vi "getLVProjBuildItems(From XML).vi"(8 "error in (no error)":errorcluster, 11 "Path":path=path "Y:/Dossiers Personnels/BRO/DevTools_BR/BuildAutomation/Builder/Builder.lvproj") -> (0 "error out":errorcluster, 1 "BuildSpec Names":string[][](array[string]), 2 "Target Names":string[](array[string]), 3 "Project Name":string, 4 "BuildSpec Types":string[][](array[string]), 5 "Project Path":path=path "Y:/Dossiers Personnels/BRO/DevTools_BR/BuildAutomation/Builder/Builder.lvproj")   [LabVIEW 2017, in "BuildServer.lvlib" / "BuildServer.lvclass"]
uses:
  BuildServer.lvclass
  <vilib>/xml/Load XML File.vi
  <vilib>/xml/Close Reference(Node).vi
  <vilib>/xml/Close Reference(NNMap).vi
  <vilib>/xml/NI_XML.lvlib
  <resource>/objmgr/DOMUserDefRef.rc
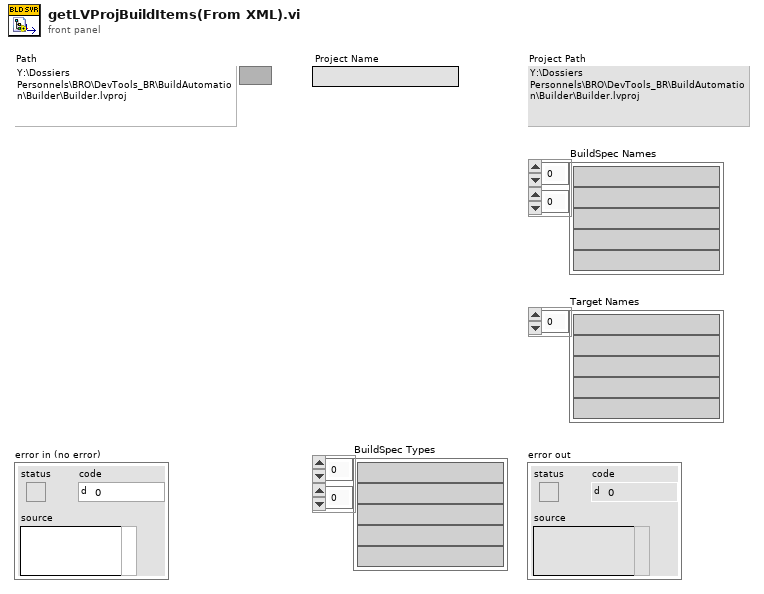
[diagram p1: front panel]
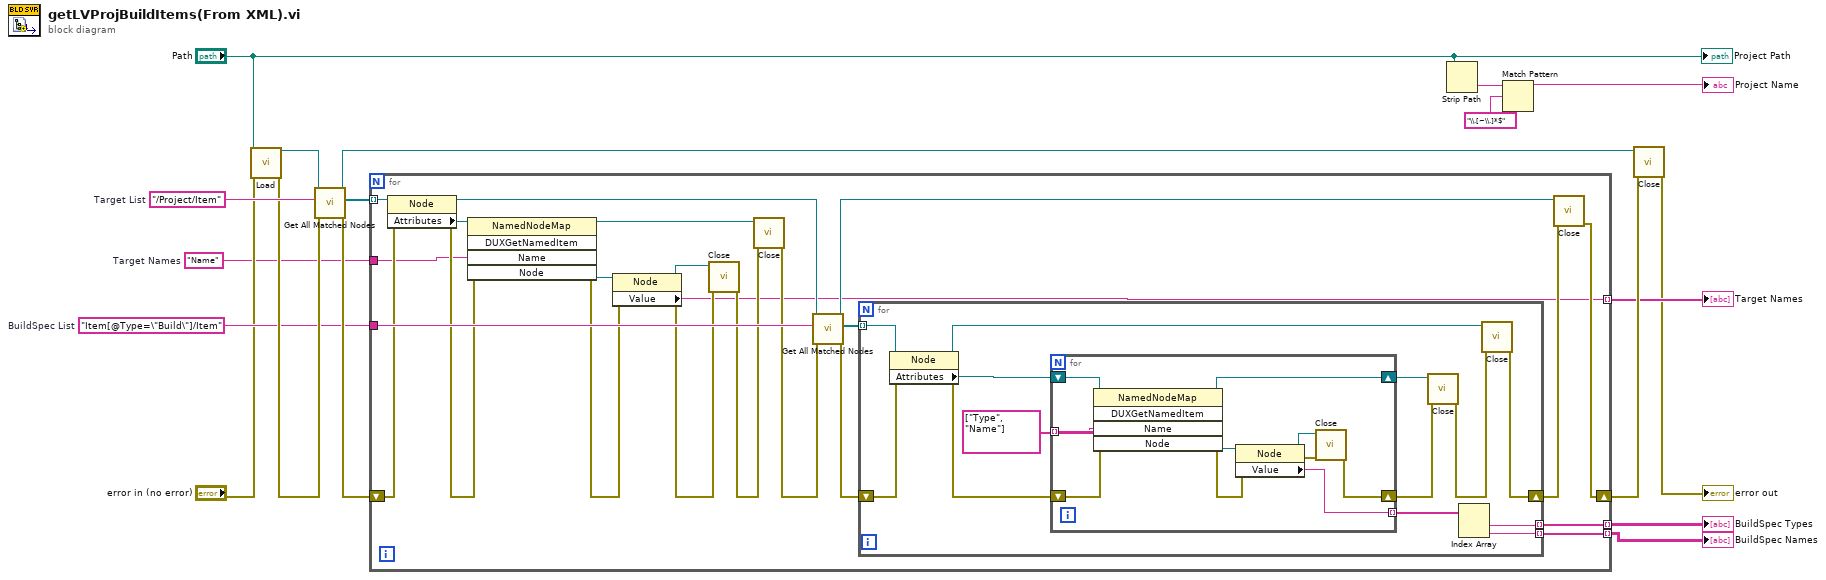
[diagram p0: block diagram]
diagram:
  w7 = "Name"  # Target Names
  w13 = "Item[@Type=\"Build\"]/Item"  # BuildSpec List
  w17 = "/Project/Item"  # Target List
  n1 = call-poly <vilib>:"Load.vi"("path to XML document"="Path", "error in (no error)"="error in (no error)") -> ("DOM document out"=w18:refnum<k20>, "error out"=w16:errorcluster)  [unwired: 11 in, 1 out]
  n2 = call <vilib>:"Get All Matched Nodes.vi"("error in (no error)"=w16, "XPath expression"=w17, "node in"=w18) -> ("error out"=w14:errorcluster, "node result array"=w15:refnum<k20>[], "node out"=w12:refnum<k20>)  [unwired: 6 in]
  n3 = for {
    tunnel: w15 -> [w34] mode=indexing
    shift-right: [w35] -> w11
    shift-left: w14 -> [w26]
    tunnel: w13 -> [w36]
    tunnel: [w22] -> w10 mode=indexing
    tunnel: w7 -> [w21]
    tunnel: [w20] -> w5 mode=indexing
    tunnel: [w19] -> w4 mode=indexing
    n4 = property class="Node"(reference=w34, error in=w26) -> (reference out=w33:refnum<k20>, error out=w27:errorcluster, "Attributes"=w32:refnum<k20>)
    n5 = invoke class="NamedNodeMap" method="DUXGetNamedItem"(reference=w32, error in=w27, "Name"=w21) -> (reference out=w25:refnum<k20>, error out=w28:errorcluster, "Node"=w31:refnum<k20>)  [unwired: 2 in, 2 out]
    n6 = property class="Node"(reference=w31, error in=w28) -> (reference out=w30:refnum<k20>, error out=w29:errorcluster, "Value"=w22:string)
    n7 = call-poly <vilib>:"Close.vi"("error in (no error)"=w29, "node"=w30) -> ("error out"=w23:errorcluster)  [unwired: 7 in]
    n8 = call-poly <vilib>:"Close.vi"("error in (no error)"=w23, "named node map"=w25) -> ("error out"=w24:errorcluster)  [unwired: 7 in]
    n9 = call <vilib>:"Get All Matched Nodes.vi"("error in (no error)"=w24, "XPath expression"=w36, "node in"=w33) -> ("error out"=w38:errorcluster, "node result array"=w39:refnum<k20>[], "node out"=w40:refnum<k20>)  [unwired: 6 in]
    n10 = for {
      tunnel: w39 -> [w49] mode=indexing
      shift-right: [w44] -> w37
      shift-left: w38 -> [w48]
      tunnel: [w42] -> w20 mode=indexing
      tunnel: [w41] -> w19 mode=indexing
      n11 = property class="Node"(reference=w49, error in=w48) -> (reference out=w53:refnum<k20>, error out=w51:errorcluster, "Attributes"=w52:refnum<k20>)
      n12 = for {
        tunnel: string[] ["Type", "Name"] -> [w62] mode=indexing
        tunnel: [w61] -> w43 mode=indexing
        shift-right: [w59] -> w47
        shift-left: w52 -> [w63]
        shift-right: [w54] -> w46
        shift-left: w51 -> [w55]
        n13 = invoke class="NamedNodeMap" method="DUXGetNamedItem"(reference=w63, error in=w55, "Name"=w62) -> (reference out=w59:refnum<k20>, error out=w56:errorcluster, "Node"=w60:refnum<k20>)  [unwired: 2 in, 2 out]
        n14 = property class="Node"(reference=w60, error in=w56) -> (reference out=w58:refnum<k20>, error out=w57:errorcluster, "Value"=w61:string)
        n15 = call-poly <vilib>:"Close.vi"("error in (no error)"=w57, "node"=w58) -> ("error out"=w54:errorcluster)  [unwired: 7 in]
      }
      n16 = call-poly <vilib>:"Close.vi"("error in (no error)"=w46, "named node map"=w47) -> ("error out"=w45:errorcluster)  [unwired: 7 in]
      n17 = Index Array(array=w43) -> (element #1=w42:string, element #2=w41:string)  [unwired: 2 in]
      n18 = call-poly <vilib>:"Close.vi"("error in (no error)"=w45, "node"=w53) -> ("error out"=w44:errorcluster)  [unwired: 7 in]
    }
    n19 = call-poly <vilib>:"Close.vi"("error in (no error)"=w37, "node"=w40) -> ("error out"=w35:errorcluster)  [unwired: 7 in]
  }
  "BuildSpec Types" <- w5
  "Target Names" <- w10
  "BuildSpec Names" <- w4
  n20 = Strip Path(path="Path") -> (name=w2:string)  [unwired: 1 out]
  n21 = Match Pattern(string=w2, regular expression="\\.[~\\.]*$") -> (before substring=→"Project Name":string)  [unwired: 4 out]
  n22 = call-poly <vilib>:"Close.vi"("error in (no error)"=w11, "node"=w12) -> ("error out"=→"error out":errorcluster)  [unwired: 7 in]
  "Project Path" <- "Path"
